vi "Read Bias Voltage Index.vi"(11 "LCR-Measurement in":refnum<class "LCR-Meas.lvclass">) -> (2 "Bias Voltage Index":i32, 3 "LCR-Measurement out":refnum<class "LCR-Meas.lvclass">)   [LabVIEW 2020, in "LCR-Meas.lvclass"]
uses:
  LCR-Meas.lvclass
  LCR-Meas.lvclass/LCR-Meas.ctl
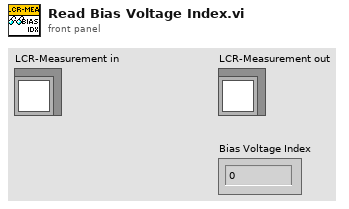
[diagram p1: front panel]
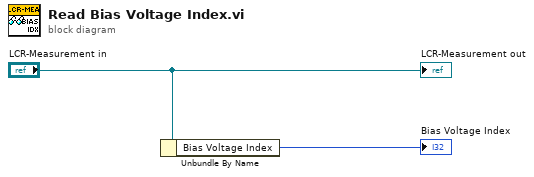
[diagram p0: block diagram]
diagram:
  n1 = Unbundle By Name("LCR-Measurement in") -> ("Bias Voltage Index"=→"Bias Voltage Index":i32)
  "LCR-Measurement out" <- "LCR-Measurement in"
